vi "Close Instrument.vi"(8 "error in (no error)":errorcluster, 11 "Ag Sig Gen.lvclass in":refnum<class "Ag Sig Gen.lvclass">) -> (0 "error out":errorcluster, 3 "Ag Sig Gen.lvclass out":refnum<class "Ag Sig Gen.lvclass">)   [LabVIEW 2010, in "Ag Sig Gen.lvclass"]
uses:
  Ag Sig Gen.lvclass
  Ag Sig Gen.lvclass/Ag Sig Gen.ctl
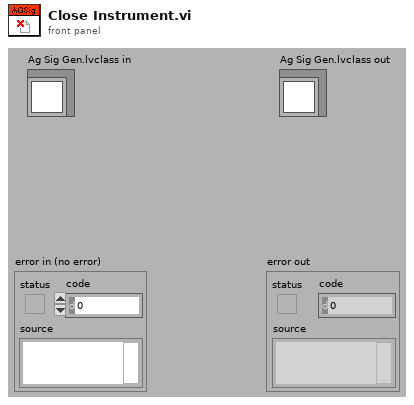
[diagram p1: front panel]
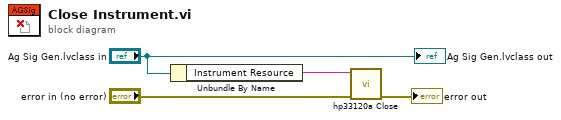
[diagram p0: block diagram]
diagram:
  n1 = Unbundle By Name("Ag Sig Gen.lvclass in") -> ("Instrument Resource"=w1:string)
  n2 = call <instrlib>:"hp33120a Close.vi"("error in (no error)"="error in (no error)", "Instrument Handle"=w1) -> ("error out"=→"error out":errorcluster)  [unwired: 9 out]
  "Ag Sig Gen.lvclass out" <- "Ag Sig Gen.lvclass in"
